vi "Scan_Limit.vi"(8 "Error In":errorcluster caption="错误输入（无错误）", 9 "扫描个数":dbl, 10 "扫描间隔(μm)":dbl, 11 "当前值(mm)":dbl) -> (0 "Error Out":errorcluster caption="错误输出", 3 "超出范围":bool)   [LabVIEW 2020]
panel:
  # "超出范围"
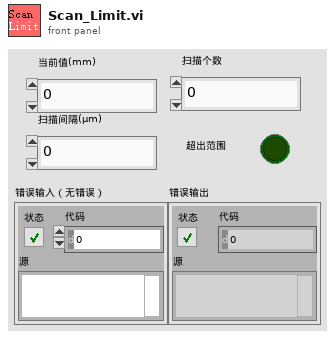
[diagram p1: front panel]
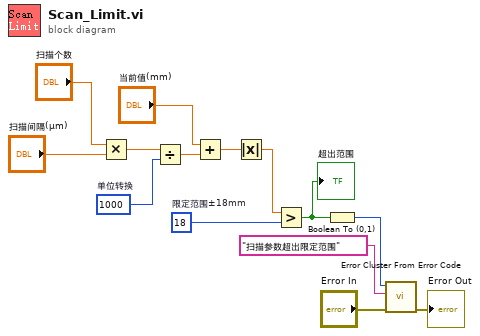
[diagram p0: block diagram]
diagram:
  w6 = 18  # 限定范围±18mm
  w12 = 1000  # 单位转换
  n1 = Multiply(x="扫描个数", y="扫描间隔(μm)") -> (x*y=w11:dbl)
  n2 = Divide(x=w11, y=w12) -> (x/y=w10:dbl)
  n3 = Add(x="当前值(mm)", y=w10) -> (x+y=w8:dbl)
  n4 = Absolute Value(x=w8) -> (abs(x)=w7:dbl)
  n5 = Greater?(x=w7, y=w6) -> (0:w5:bool)
  "超出范围" <- w5
  n6 = Boolean To (0,1)(Boolean=w5) -> (0, 1=w4:i16)
  n7 = call <vilib>:"Error Cluster From Error Code.vi"("error in (no error)"="Error In", "error message (\"\")"="扫描参数超出限定范围", "error code (0)"=w4) -> ("error out"=→"Error Out":errorcluster)  [unwired: 6 in]
